vi "SaveTuneOld.vi"(0 "Array":dbl[](array[numeric]), 1 "Save Data to File":bool, 2 "Ext time (sec)":dbl format="%#_10g") -> (3 "Current time (sec)":dbl format="%#_10g")   [LabVIEW 2018]
uses:
  Global 2.vi
  kleinjan/MKS/Global - Pressure & Flow.vi
  <vilib>/Utility/file.llb/Write To Spreadsheet File (string).vi
  <vilib>/Utility/file.llb/Write To Spreadsheet File (DBL).vi
panel:
  out "Appended array":dbl[](array[numeric]) format="%#_10g"
  out "File name":string
  # "Saves data to spreadsheet file"
  # "Creates file with name including current time\nand header plus data"
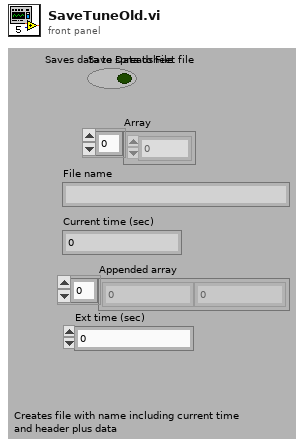
[diagram p1: front panel]
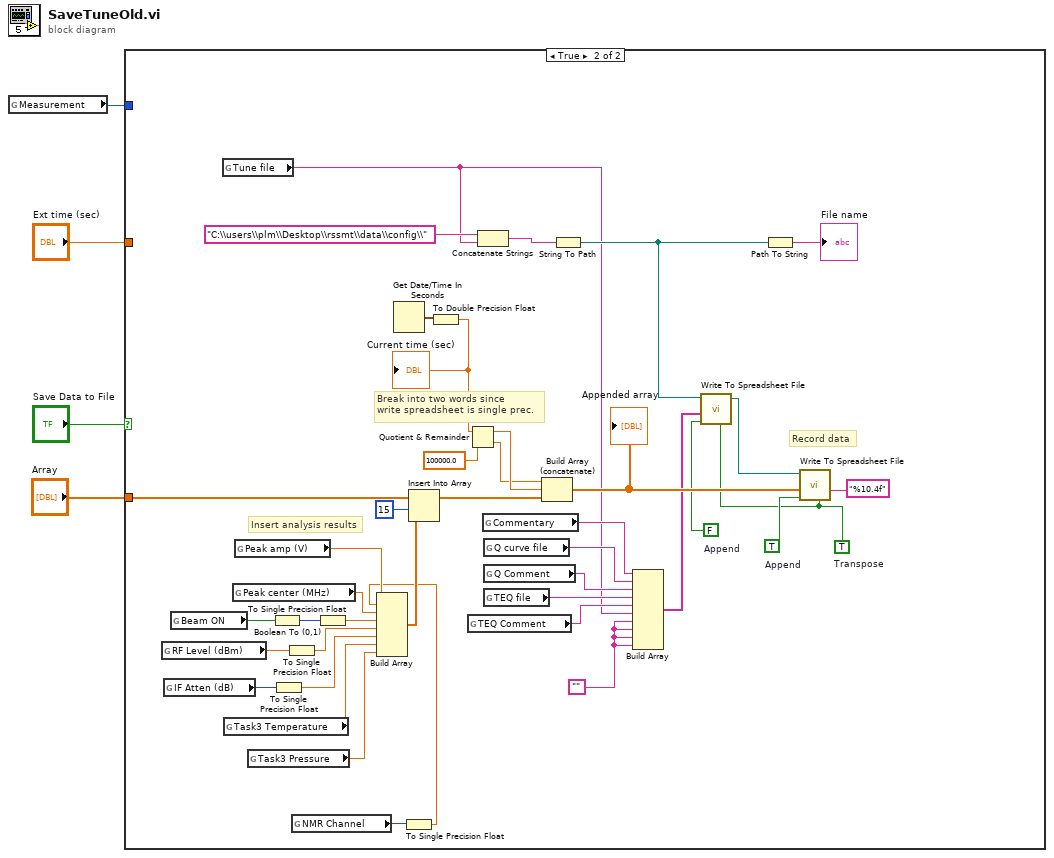
[diagram p0: block diagram]
diagram:
  n1 = global read "Global 2.vi" "Measurement"() -> (w1:enum16{"TEQ", "POL", "QCV"})
  n2 = case shown="True" "Save Data to File" {
    tunnel: "Array" -> [_ w25]
    tunnel: "Ext time (sec)" -> [_ _]
    tunnel: w1 -> [_ _]
    frame False {
      # "Not writing file"
    }
    frame True {
      w5 = FALSE  # Append
      w19 = ""
      w31 = TRUE  # Append
      w30 = TRUE  # Transpose
      # "Insert analysis results"
      # "Record data"
      # "Break into two words since\nwrite spreadsheet is single prec."
      n3 = global read "Global 2.vi" "RF Level (dBm)"() -> (w13:dbl)
      n4 = global read "Global 2.vi" "IF Atten (dB)"() -> (w11:i8)
      n5 = global read "Global 2.vi" "Beam ON"() -> (w15:bool)
      n6 = global read "Global 2.vi" "Tune file"() -> (w6:string)
      n7 = global read "Global - Pressure & Flow.vi" "Task3 Temperature"() -> (w9:dbl)
      n8 = global read "Global 2.vi" "Peak center (MHz)"() -> (w20:sgl)
      n9 = global read "Global 2.vi" "Peak amp (V)"() -> (w22:sgl)
      n10 = global read "Global - Pressure & Flow.vi" "Task3 Pressure"() -> (w8:dbl)
      n11 = Boolean To (0,1)(Boolean=w15) -> (0, 1=w16:i16)
      n12 = To Single Precision Float(number=w11) -> (single precision float=w10:sgl)
      n13 = To Single Precision Float(number=w13) -> (single precision float=w12:sgl)
      n14 = global read "Global 2.vi" "NMR Channel"() -> (w18:i32)
      n15 = To Single Precision Float(number=w16) -> (single precision float=w14:sgl)
      n16 = Get Date/Time In Seconds() -> (seconds since 1Jan1904=w42:timestamp)
      n17 = To Single Precision Float(number=w18) -> (single precision float=w17:sgl)
      n18 = Build Array(w22, w17, w20, w14, w12, w10, w9, w8) -> (w21:dbl[])
      n19 = Insert Into Array "Insert Into Array"(array=w25, index=15, new element=w21) -> (w24:dbl[])
      n20 = To Double Precision Float(number=w42) -> (double precision float=w40:dbl)
      "Current time (sec)" <- w40
      n21 = Quotient & Remainder(x=w40, y=100000.0) -> (x-y*floor(x/y)=w39:dbl, floor(x/y)=w37:dbl)
      n22 = global read "Global 2.vi" "TEQ Comment"() -> (w27:string)
      n23 = Concatenate Strings("C:\\users\\plm\\Desktop\\rssmt\\data\\config\\", w6) -> (w44:string)
      n24 = global read "Global 2.vi" "Commentary"() -> (w33:string)
      n25 = global read "Global 2.vi" "Q curve file"() -> (w29:string)
      n26 = global read "Global 2.vi" "Q Comment"() -> (w28:string)
      n27 = global read "Global 2.vi" "TEQ file"() -> (w26:string)
      n28 = Build Array (concatenate) "Build Array"(w37, w39, w24) -> (w41:dbl[])
      "Appended array" <- w41
      n29 = String To Path(string=w44) -> (path=w35:path)
      n30 = Build Array(w33, w29, w28, w26, w27, w6, w19, w19, w19, w19) -> (w32:string[])
      n31 = call-poly <vilib>:"Write To Spreadsheet File.vi"("transpose? (no:F)"=w30, "append to file? (new file:F)"=w5, "1D data"=w32, "file path (dialog if empty)"=w35) -> ("new file path (Not A Path if cancelled)"=w34:path)  [unwired: 4 in]
      n32 = Path To String(path=w35) -> (string=→"File name":string)
      n33 = call-poly <vilib>:"Write To Spreadsheet File.vi"("transpose? (no:F)"=w30, "format (%.3f)"="%10.4f", "append to file? (new file:F)"=w31, "1D data"=w41, "file path (dialog if empty)"=w34) -> ()  [unwired: 3 in, 1 out]
    }
  }
